vi "Unflatten_ClassGen.vi"(8 "error in (no error)":errorcluster caption="entrée d'erreur (pas d'erreur)", 11 "XML File Path":path caption="Chemin du fichier XML") -> (0 "sortie d'erreur":errorcluster, 3 "LabVIEW Object":refnum<class>)   [LabVIEW 2019]
uses:
  <vilib>/Utility/xml.llb/Read From XML File(string).vi
panel:
  out "Flattened Class XML String":string
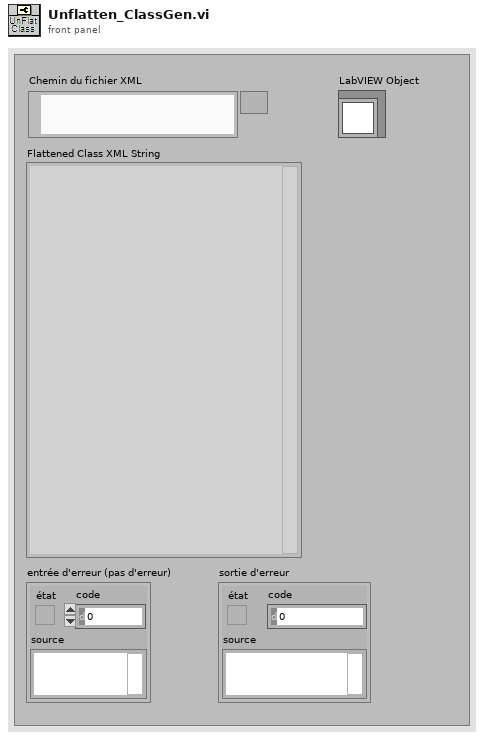
[diagram p1: front panel]
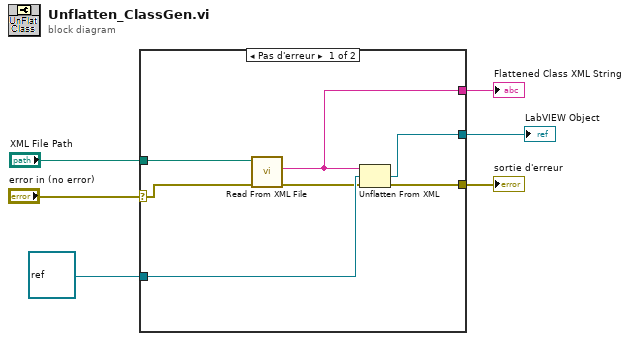
[diagram p0: block diagram]
diagram:
  n1 = case shown="Pas d'erreur" "error in (no error)" {
    selector: "error in (no error)" -> [w11 w15]
    tunnel: refnum<class> refnum ("LabVIEW Object") -> [w13 w14]
    tunnel: "XML File Path" -> [w12 _]
    tunnel: [w9 w15] -> w4
    tunnel: [w8 w14] -> w1
    tunnel: [w7 _] -> w3
    frame No Error {
      n2 = call-poly <vilib>:"Read From XML File.vi"("error in (no error)"=w11, "XML File Path"=w12) -> ("error out"=w10:errorcluster, "XML Elements"=w7:string)  [unwired: 7 in, 1 out]
      n3 = Unflatten From XML(xml string=w7, type=w13, error in (no error)=w10) -> (value=w8:refnum<class>, error out=w9:errorcluster)
    }
    frame Error {
    }
  }
  "Flattened Class XML String" <- w3
  "sortie d'erreur" <- w4
  "LabVIEW Object" <- w1
